vi "SetAdGain.vi"(1 "gain":u8=6) -> ()   [LabVIEW 2015]
uses:
  ESLSCDLL.dll
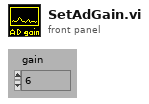
[diagram p1: front panel]
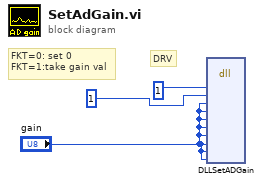
[diagram p0: block diagram]
diagram:
  # "FKT=0: set 0\nFKT=1:take gain val"
  # "DRV"
  n1 = dll-call lib="C:/ENTW/PCIE/64bit/lv64/1cam/board.vis/ESLSCDLL.dll" fn="DLLSetADGain" ("lwlscdll.dll:DLLSetADAmpRed")("drv"=u32 1, "fkt"=u8 1, "g1"="gain", "g2"="gain", "g3"="gain", "g4"="gain", "g5"="gain", "g6"="gain", "g7"="gain", "g8"="gain") -> ()  [unwired: 14 in, 2 out]
